vi "WorkingI2C.vi"   [LabVIEW 2015]
uses:
  <vilib>/Aledyne-TSXperts/Arduino Compatible Compiler for LabVIEW/Code Generator/Arduino APIs/Serial/Serial Settings.ctl
  <vilib>/Aledyne-TSXperts/Arduino Compatible Compiler for LabVIEW/Code Generator/Arduino APIs/I2C/I2C Mode.ctl
  <vilib>/Aledyne-TSXperts/Arduino Compatible Compiler for LabVIEW/Arduino Compatible Compiler for LabVIEW.lvlib
types:
  T1 = typedef "Arduino Compatible Compiler for LabVIEW.lvlib/I2C Mode.ctl" = enum16{"Master", "Slave"}
  T2 = typedef "Arduino Compatible Compiler for LabVIEW.lvlib/Serial Settings.ctl" = u16
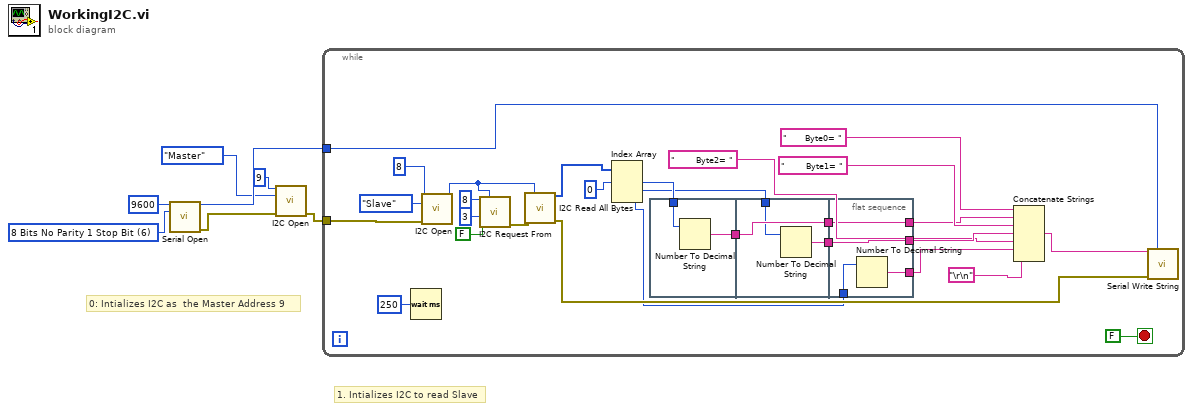
[diagram p0: block diagram]
diagram:
  w7 = T2 6 items=["5 Bits No Parity 1 Stop Bit"=0, "6 Bits No Parity 1 Stop Bit"=2, "7 Bits No Parity 1 Stop Bit"=4, "8 Bits No Parity 1 Stop Bit"=6, "5 Bits No Parity 2 Stop Bits"=8, "6 Bits No Parity 2 Stop Bits"=10, "7 Bits No Parity 2 Stop Bits"=12, "8 Bits No Parity 2 Stop Bits"=14, "5 Bits Even Parity 1 Stop Bits"=32, "6 Bits Even Parity 1 Stop Bits"=34, "7 Bits Even Parity 1 Stop Bits"=36, "8 Bits Even Parity 1 Stop Bits"=38, "5 Bits Even Parity 2 Stop Bits"=40, "6 Bits Even Parity 2 Stop Bits"=42, "7 Bits Even Parity 2 Stop Bits"=44, "8 Bits Even Parity 2 Stop Bits"=46, "5 Bits Odd Parity 1 Stop Bits"=48, "6 Bits Odd Parity 1 Stop Bits"=50, "7 Bits Odd Parity 1 Stop Bits"=52, "8 Bits Odd Parity 1 Stop Bits"=54, "5 Bits Odd Parity 2 Stop Bits"=56, "6 Bits Odd Parity 2 Stop Bits"=58, "7 Bits Odd Parity 2 Stop Bits"=60, "8 Bits Odd Parity 2 Stop Bits"=62] ("Serial Settings")
  # "1. Intializes I2C to read Slave"
  # "0: Intializes I2C as  the Master Address 9"
  n1 = call <vilib>:"Serial Open.vi"("Speed"=u32 9600, "Serial Settings"=w7) -> ("Instance"=w5:u8, "error out"=w3:errorcluster)  [unwired: 12 in]
  n2 = call <vilib>:"I2C Open.vi"("Slave Address"=u8 9, "Mode"=I2C_Mode."Master", "error in (no error)"=w3) -> ("error out"=w2:errorcluster)  [unwired: 11 in, 1 out]
  n3 = while {
    tunnel: w5 -> [w26]
    tunnel: w2 -> [w25]
    stop <- FALSE stop-if-true
    n4 = Wait (ms)(milliseconds to wait=u32 250) -> ()  [unwired: 1 out]
    n5 = call <vilib>:"I2C Open.vi"("Slave Address"=u8 8, "Mode"=I2C_Mode."Slave", "error in (no error)"=w25) -> ("Interface"=w14:u8)  [unwired: 11 in, 1 out]
    n6 = call <vilib>:"I2C Request From.vi"("Slave Address"=u8 8, "Interface"=w14, "Number of Bytes"=u32 3, "Send Stop"=FALSE) -> ("error out"=w18:errorcluster)  [unwired: 11 in]
    n7 = call <vilib>:"I2C Read All Bytes.vi"("Interface"=w14, "error in (no error)"=w18) -> ("Data"=w22:u8[], "error out"=w21:errorcluster)  [unwired: 12 in]
    n8 = Index Array(array=w22, index #1=0 ("index")) -> (element #1=w20:u8, element #2=w19:u8, element #3=w10:u8)  [unwired: 2 in]
    n9 = flat-sequence {
      tunnel: [w37] -> w34
      tunnel: w20 -> [w36]
      tunnel: w34 -> [w40]
      tunnel: w19 -> [w38]
      tunnel: [w40] -> w12
      tunnel: [w39] -> w11
      tunnel: [w43] -> w30
      tunnel: [w44] -> w28
      tunnel: w12 -> [w44]
      tunnel: w11 -> [w43]
      tunnel: w10 -> [w42]
      tunnel: [w41] -> w9
      frame #0 {
        n10 = Number To Decimal String(number=w36) -> (decimal integer string=w37:string)  [unwired: 1 in]
      }
      frame #1 {
        n11 = Number To Decimal String(number=w38) -> (decimal integer string=w39:string)  [unwired: 1 in]
      }
      frame #2 {
        n12 = Number To Decimal String(number=w42) -> (decimal integer string=w41:string)  [unwired: 1 in]
      }
    }
    n13 = Concatenate Strings("      Byte0= " ("String"), w28, "       Byte1= " ("String"), w30, "       Byte2= " ("String"), w9, "\r\n" ("End of Line Constant")) -> (w32:string)
    n14 = call <vilib>:"Serial Write String.vi"("String"=w32, "Instance"=w26, "error in (no error)"=w21) -> ()  [unwired: 12 in, 1 out]
  }
